vi "check_attribute.vi"(6 "Access":enum16{"Read", "Write"}(ring)=enum."Write", 7 "Attribute":T2={"Identifier"="", "Descriptive name"="", "Data Type"=enum."Integer 32", "Command"="", "Access"=2, "Range Table"="", "Read Callback"="", "Write Callback"="", "Range Callback"="", "Check Callback"="", "Rngtable Callback"="", "Coerce Callback"="", "Supported Models"="", "Instrument Options"="", "Repeated Capabilities"="", "Check Status Callback"="", "Index"=0, "Flag: OPC Wait"=FALSE, "Flag: Dont check status"=FALSE, "Flag: Cache Only"=FALSE} {"Access" items=["Read Only", "Write Only", "Read/Write"]}, 8 "error in":errorcluster, 10 "Data Type":T1, 11 "VISA resource name":refnum<visa-resource-name>) -> (0 "error out":errorcluster, 3 "VISA resource name out":refnum<visa-resource-name>)   [LabVIEW 2014, in "rszvl_rsidr_core.lvlib"]
uses:
  rszvl_rsidr_core.lvlib
  type_Attribute.ctl
  type_Attribute_Data_Type.ctl
  type_Error_Codes.ctl
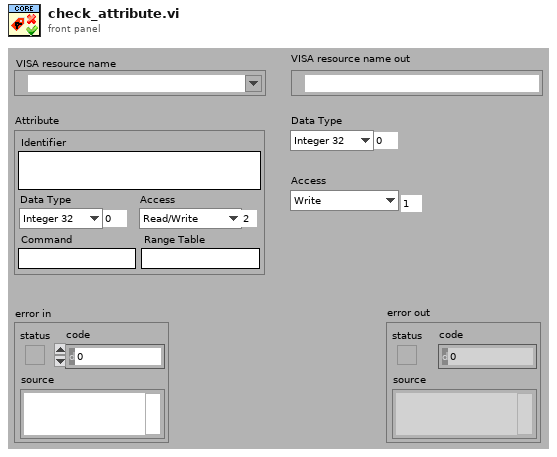
[diagram p1: front panel]
types:
  T1 = typedef "rszvl_rsidr_core.lvlib/type_Attribute_Data_Type.ctl" = enum16{"Integer 32", "Double", "String", "Boolean", "None", "Integer 64"}
  T2 = typedef "rszvl_rsidr_core.lvlib/type_Attribute.ctl" = cluster{"Identifier":string, "Descriptive name":string, "Data Type":T1, "Command":string, "Access":u16, "Range Table":string, "Read Callback":string, "Write Callback":string, "Range Callback":string, "Check Callback":string, "Rngtable Callback":string, "Coerce Callback":string, "Supported Models":string, "Instrument Options":string, "Repeated Capabilities":string, "Check Status Callback":string, "Index":i32, "Flag: OPC Wait":bool, "Flag: Dont check status":bool, "Flag: Cache Only":bool}
  T3 = typedef "rszvl_rsidr_core.lvlib/type_Error_Codes.ctl" = enum16{"No_error", "VISA_err_ResourceNotFound", "VISA_err_Timeout", "VISA_warn_MoreDataAvailable", "RS_err_MissingCallback", "RS_err_InvalidAttribute", "RS_err_InvalidValue", "RS_err_UnknownResource", "RS_err_AlreadyInitialized", "RS_err_InstrumentStatus", "RS_err_BadRepCapName", "RS_err_TypesMismatch", "RS_err_ValueNotSupported", "RS_err_InvalidRngTable", "RS_err_IDqueryFail", "RS_err_UnexpResponse", "VISA_warn_ConfigNotLoaded", "RS_err_AttributeNotReadable", "RS_err_AttributeNotWritable", "RS_err_InstrumentType", "RS_err_InstrumentOption", "VISA_err_InvalidSize", "RS_err_ReliabilityIndicator", "VISA_warn_UnknownStatus", "VISA_warn_TermCharRead", "VISA_err_IO_error"}
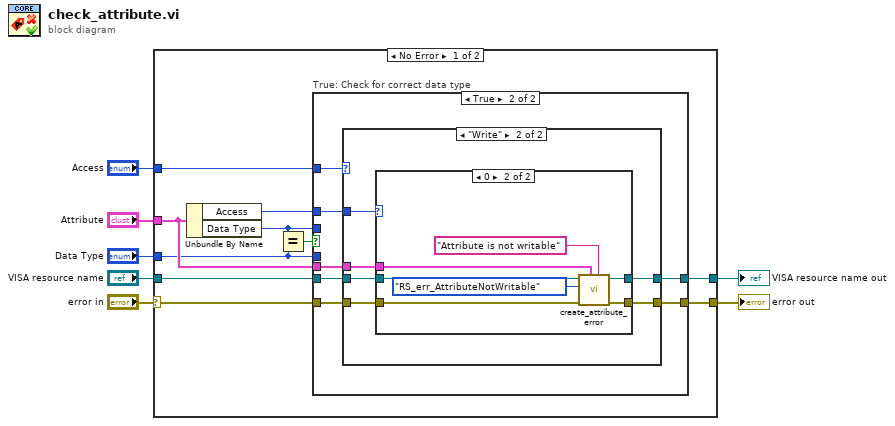
[diagram p0: block diagram]
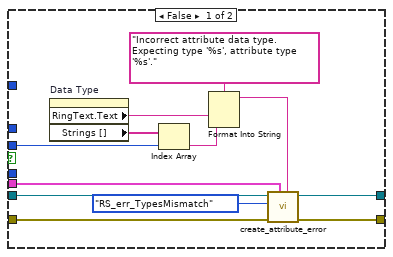
[diagram p2: hidden frame]
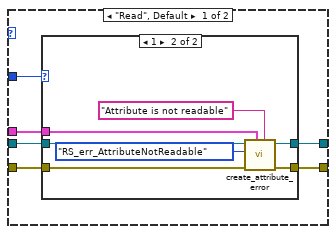
[diagram p3: hidden frame]
diagram:
  n1 = case shown="No Error" "error in" {
    selector: "error in" -> [w14 w68]
    tunnel: [w16 w68] -> w6
    tunnel: "VISA resource name" -> [w12 w67]
    tunnel: [w11 w67] -> w4
    tunnel: "Access" -> [w10 _]
    tunnel: "Attribute" -> [w9 _]
    tunnel: "Data Type" -> [w8 _]
    frame No Error {
      n2 = Unbundle By Name(w9) -> ("Access"=w15:u16, "Data Type"=w13:T1)
      n3 = Equal?(x=w13, y=w8) -> (x = y?=w17:bool)
      n4 = case "True: Check for correct data type" shown="True" w17 {
        tunnel: [w29 w34] -> w16
        tunnel: w10 -> [_ w36]
        tunnel: w15 -> [_ w35]
        tunnel: w14 -> [w28 w33]
        tunnel: w9 -> [w21 w32]
        tunnel: w8 -> [_ _]
        tunnel: w13 -> [w25 _]
        tunnel: w12 -> [w20 w30]
        tunnel: [w18 w31] -> w11
        frame False {
          n5 = property on="Data Type" class="Enum (strict)"() -> ("RingText.Text"=w27:string, "Strings []"=w26:string[])  [unwired: 2 in, 2 out]
          n6 = Index Array(array=w26, index=w25) -> (element=w23:string)
          n7 = Format Into String(format string="Incorrect attribute data type. Expecting type '%s', attribute type '%s'.", w27, w23) -> (resulting string=w22:string)  [unwired: 2 in, 1 out]
          n8 = call "create_attribute_error.vi"("Error Elaboration (\"\")"=w22, "Attribute"=w21, "error in"=w28, "Error Enum in"=type_Error_Codes."RS_err_TypesMismatch" ("Error Enum in (from err to recompose)"), "VISA resource name"=w20) -> ("error out"=w29:errorcluster, "VISA resource name out"=w18:refnum<visa-resource-name>)  [unwired: 5 in]
        }
        frame True {
          n9 = case shown="\"Write\"" w36 {
            tunnel: w35 -> [w39 w54]
            tunnel: [w42 w57] -> w34
            tunnel: w33 -> [w41 w56]
            tunnel: w32 -> [w40 w55]
            tunnel: [w38 w53] -> w31
            tunnel: w30 -> [w37 w52]
            frame "Read", Default {
              n10 = case shown="1" w39 {
                tunnel: [w44 w51] -> w42
                tunnel: w41 -> [w44 w50]
                tunnel: w40 -> [_ w49]
                tunnel: [w43 w48] -> w38
                tunnel: w37 -> [w43 w45]
                frame 0, Default {
                }
                frame 1 {
                  n11 = call "create_attribute_error.vi"("Error Elaboration (\"\")"="Attribute is not readable" ("string"), "Attribute"=w49, "error in"=w50, "Error Enum in"=type_Error_Codes."RS_err_AttributeNotReadable" ("Error Enum in (from err to recompose)"), "VISA resource name"=w45) -> ("error out"=w51:errorcluster, "VISA resource name out"=w48:refnum<visa-resource-name>)  [unwired: 5 in]
                }
              }
            }
            frame "Write" {
              n12 = case shown="0" w54 {
                tunnel: [w59 w66] -> w57
                tunnel: w56 -> [w59 w65]
                tunnel: w55 -> [_ w64]
                tunnel: [w58 w63] -> w53
                tunnel: w52 -> [w58 w62]
                frame 1, Default {
                }
                frame 0 {
                  n13 = call "create_attribute_error.vi"("Error Elaboration (\"\")"="Attribute is not writable" ("string"), "Attribute"=w64, "error in"=w65, "Error Enum in"=type_Error_Codes."RS_err_AttributeNotWritable" ("Error Enum in (from err to recompose)"), "VISA resource name"=w62) -> ("error out"=w66:errorcluster, "VISA resource name out"=w63:refnum<visa-resource-name>)  [unwired: 5 in]
                }
              }
            }
          }
        }
      }
    }
    frame Error {
    }
  }
  "VISA resource name out" <- w4
  "error out" <- w6
